vi "Main.vi"(0 "Operations":string(combo), 1 "Delete":bool, 2 "Save":bool, 3 "Load":bool, 5 "Add":bool, 7 "Tree":string(tree), 11 "Error In":errorcluster) -> (15 "Error Out":errorcluster)   [LabVIEW 2023]
doc: "The VI adds the selected the operation into the tree and loads the instances which performs the arithmetic operations and it can save or load the class data into the XML files"
uses:
  Typedef/Queue Operation.ctl
  Typedef/Calculator Data.ctl
  Typedef/Class Data.ctl
  Classes/Arithemtic Operation/Arithemetic Operation.lvclass
  Typedef/DVR Ref.ctl
  Typedef/User Event Operations.ctl
  <vilib>/Utility/xml.llb/Write to XML File(string).vi
  <vilib>/Utility/xml.llb/Read From XML File(array).vi
panel:
  # "Instructions:\n1. Run the VI.\n2. Select the operation to be done from the Operations.\n3. Click Add to create a instance and is added in the tree.\n4. Select the instance name in the tree to load the instance.\n5. Specify the input values in the instance and observe the output\n6. On clicking the Delete button the selected instance will be deleted. \n7. Click Save to save the values all instances in an XML file.\n8. Click Load to load the values of all instances from an XML file.\n9. Click panel close to stop the VI from running."
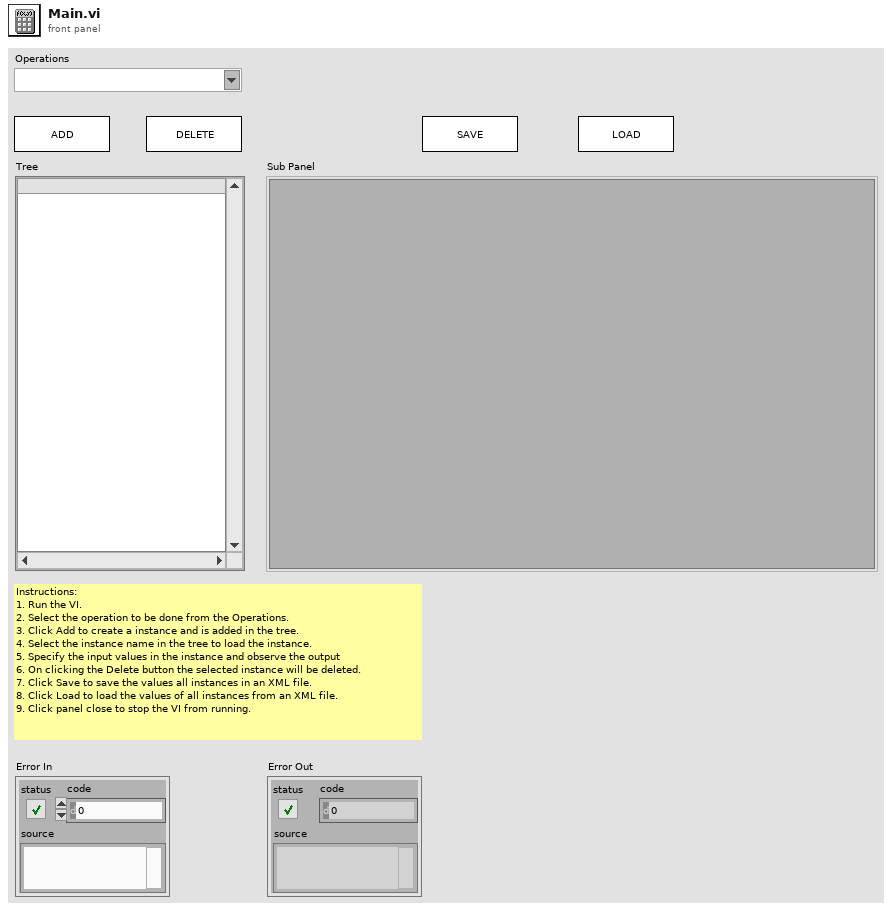
[diagram p1: front panel]
types:
  T1 = typedef "User Event Operations.ctl" = enum16{"Obtain", "Generate", "Release"}
  T2 = typedef "Calculator Data.ctl" = cluster{"Selected Item":string, "Selected Tag":string, "XML Path":path, "Instance Data Array":T3[], "Class Data":refnum<class "Arithemetic Operation.lvclass">, "Class Name":string, "Close":refnum<data-value>, "DVR Ref Array":T4[]}
  T3 = typedef "Class Data.ctl" = cluster{"Class Data":refnum<class "Arithemetic Operation.lvclass">, "Name":string}
  T4 = typedef "DVR Ref.ctl" = cluster{"Class Name":string, "DVR":refnum<data-value>}
  T5 = typedef "Queue Operation.ctl" = enum16{"Create & Enqueue N", "Enqueue N", "Dequeue", "Enstack N", "Flush", "Release"}
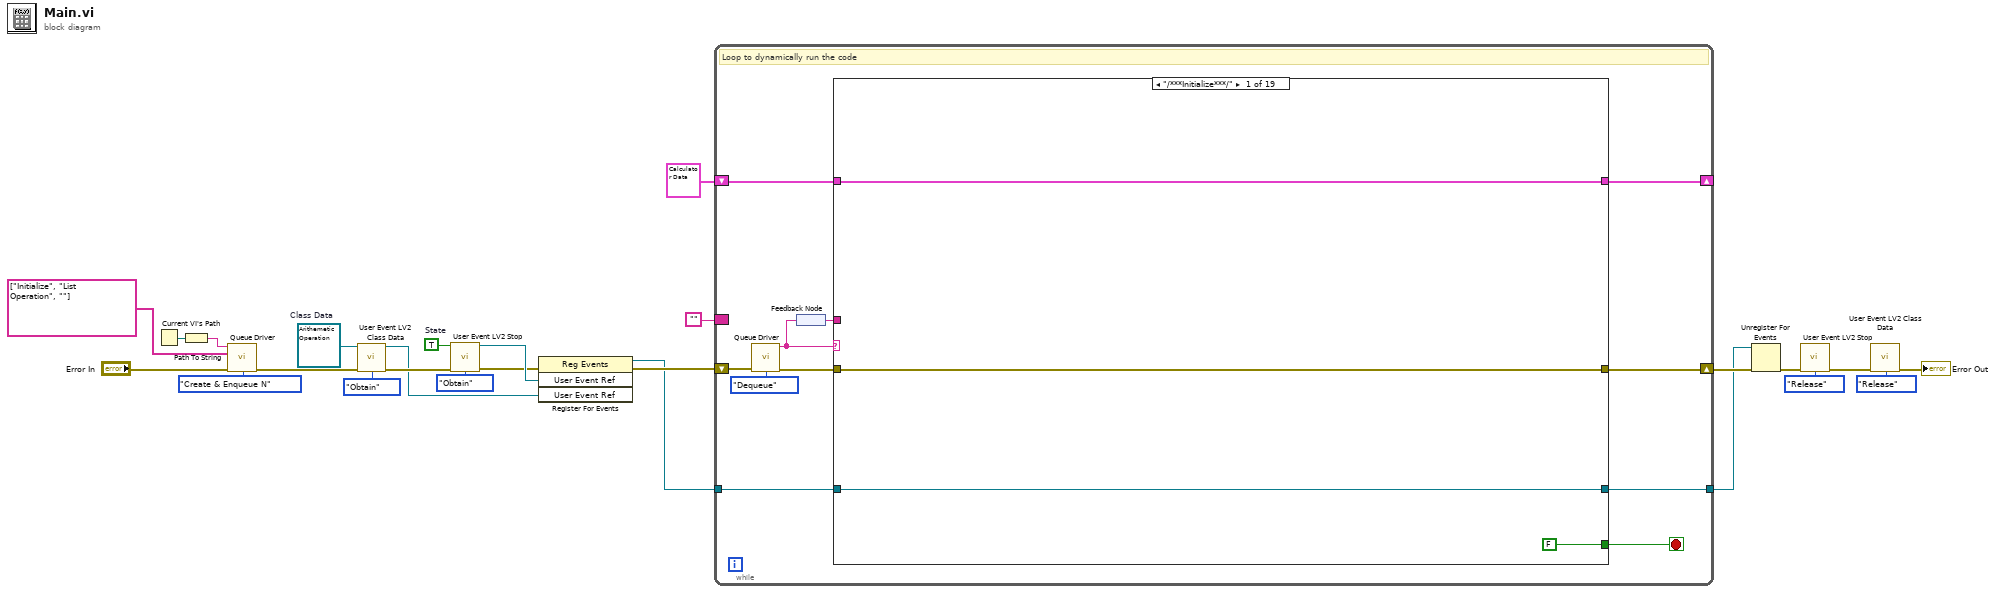
[diagram p0: block diagram]
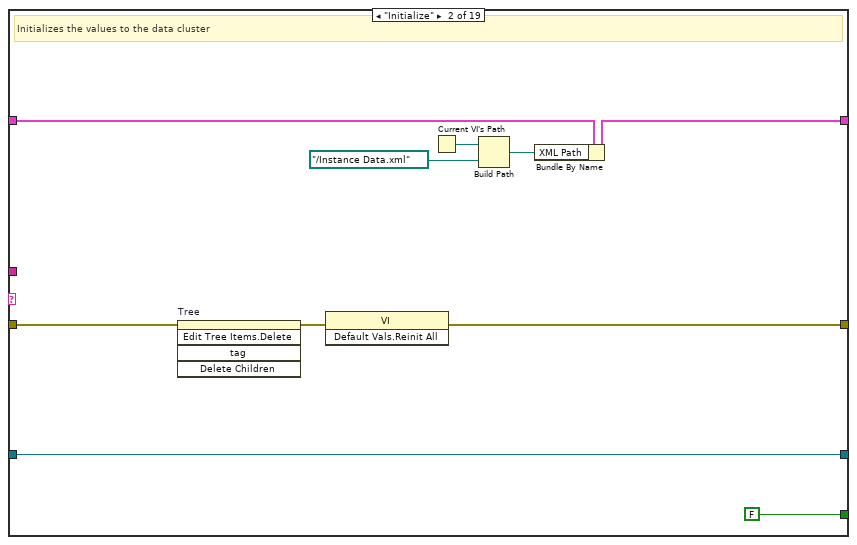
[diagram p2: hidden frame]
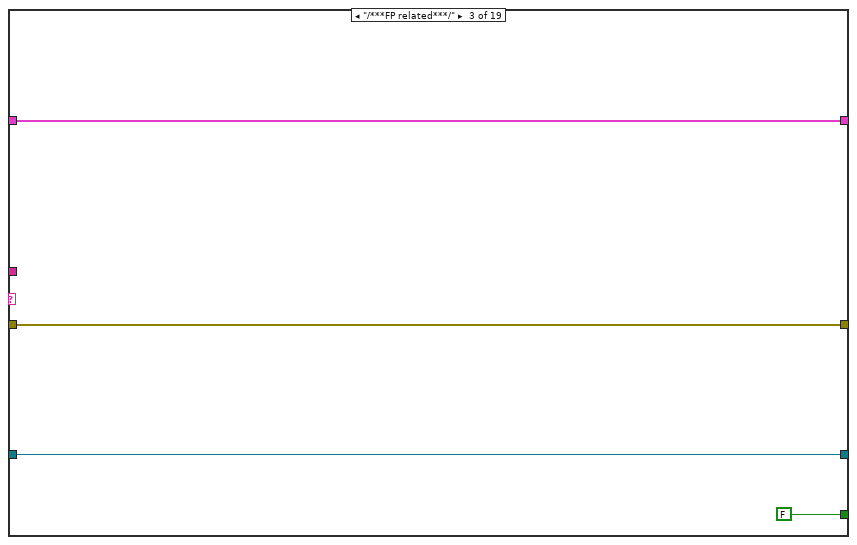
[diagram p3: hidden frame]
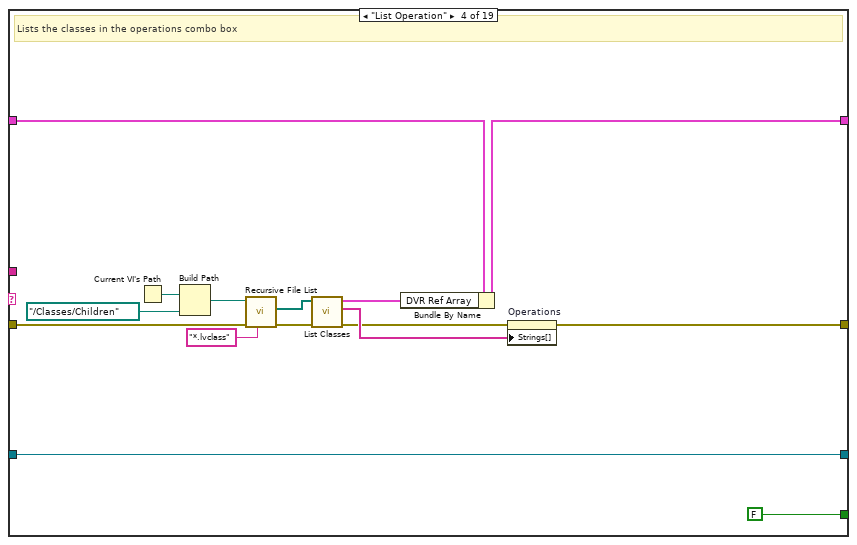
[diagram p4: hidden frame]
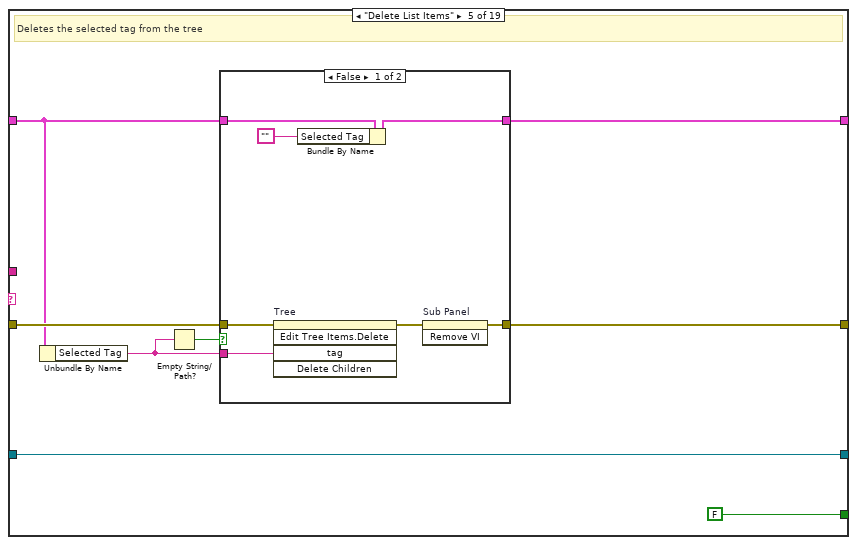
[diagram p5: hidden frame]
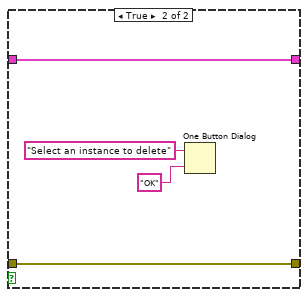
[diagram p6: hidden frame]
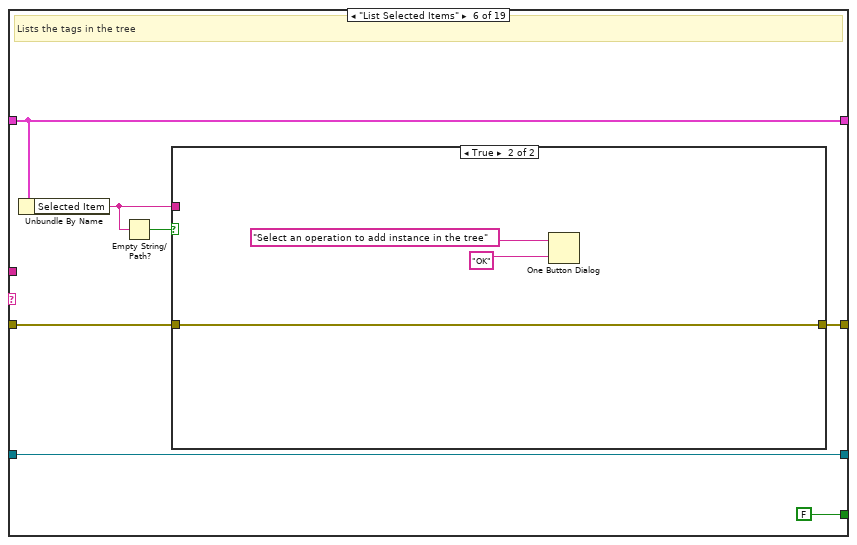
[diagram p7: hidden frame]
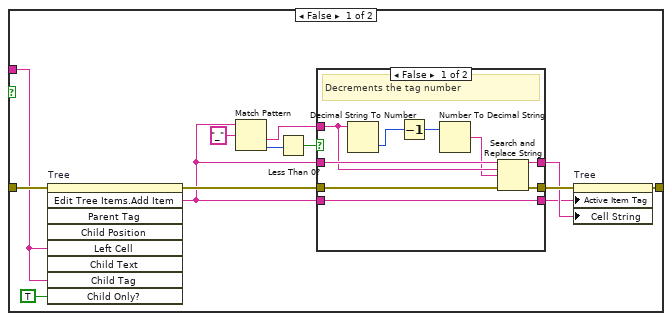
[diagram p8: hidden frame]
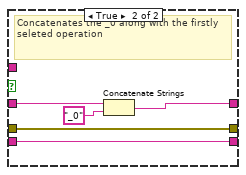
[diagram p9: hidden frame]
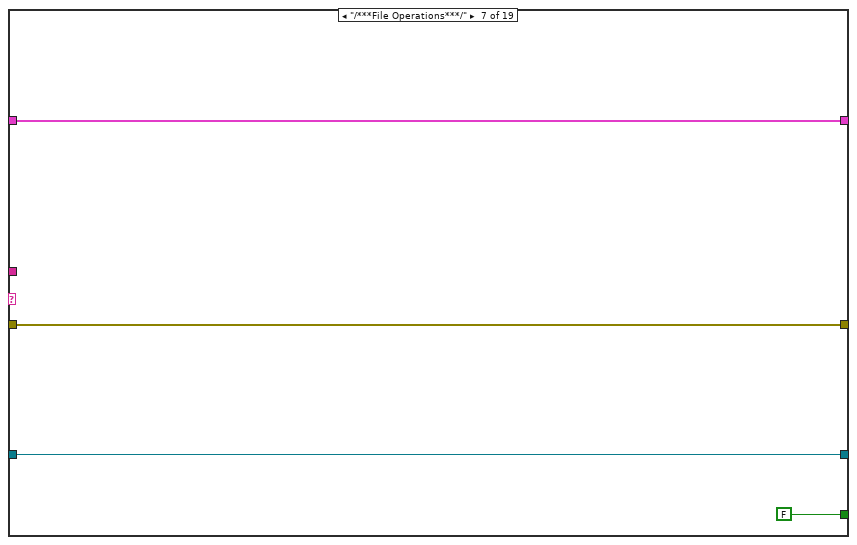
[diagram p10: hidden frame]
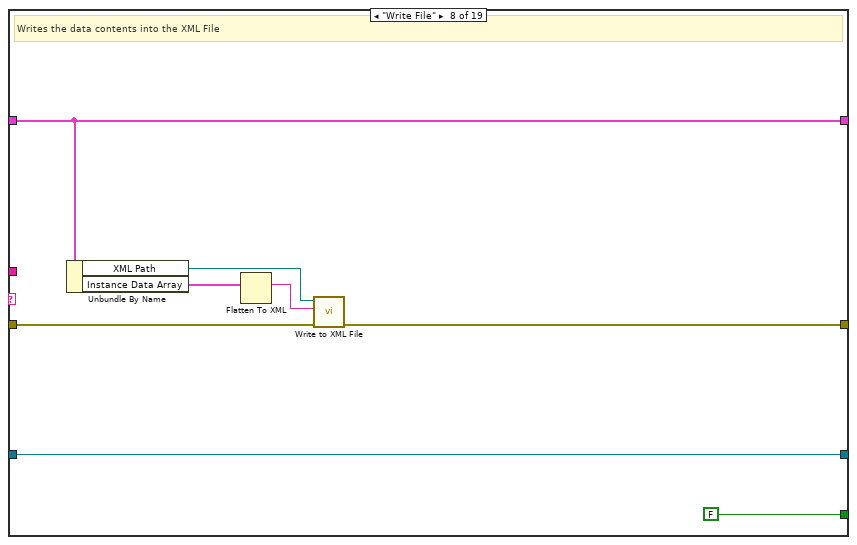
[diagram p11: hidden frame]
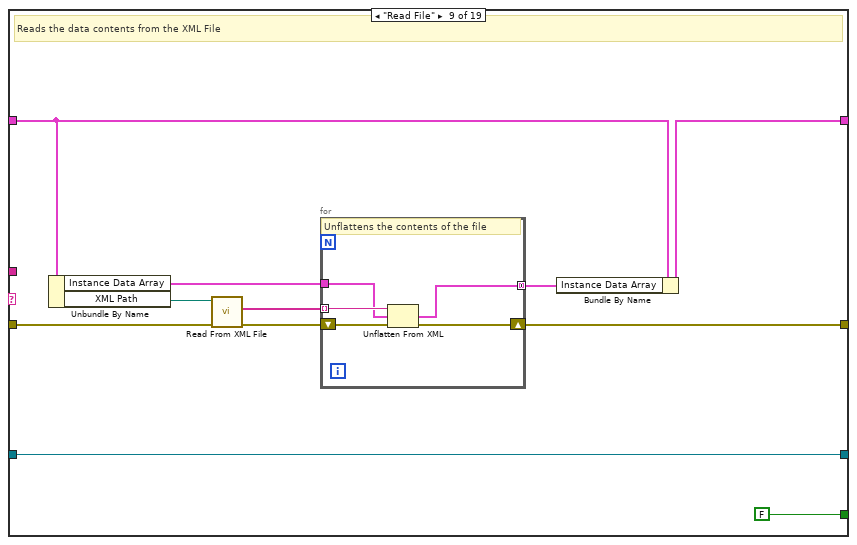
[diagram p12: hidden frame]
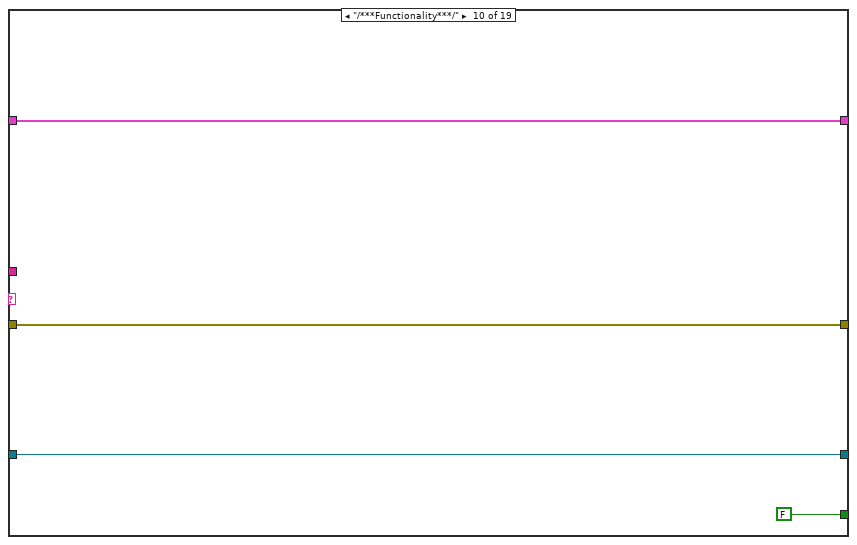
[diagram p13: hidden frame]
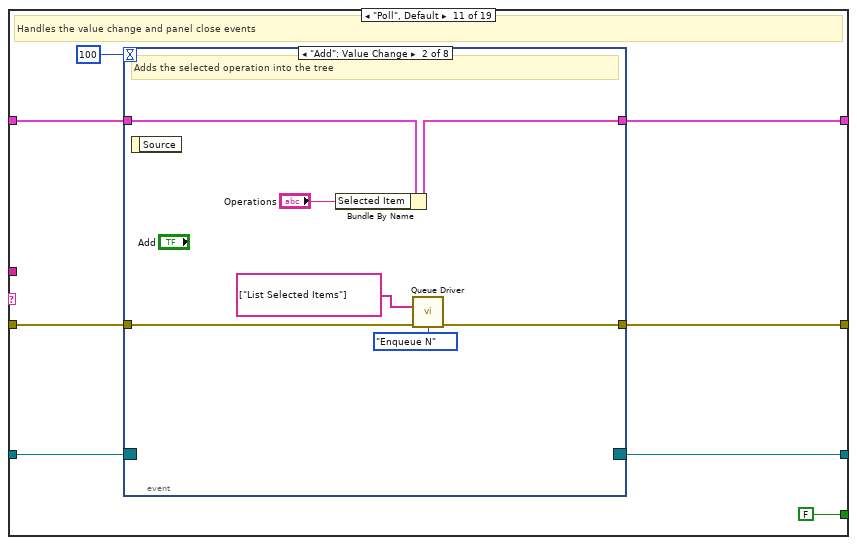
[diagram p14: hidden frame]
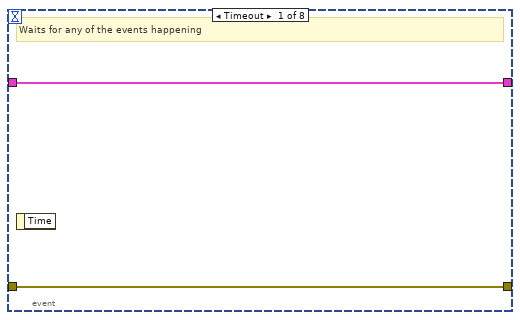
[diagram p15: hidden frame]
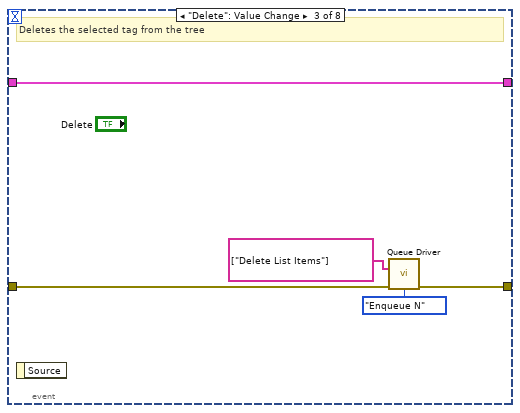
[diagram p16: hidden frame]
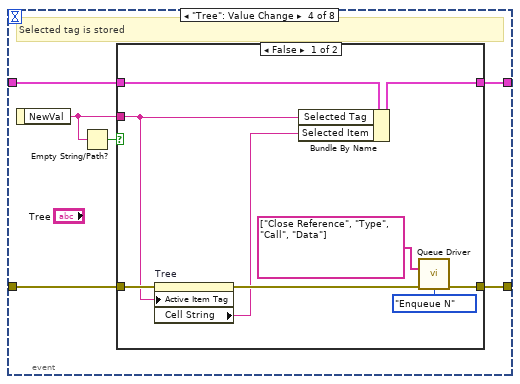
[diagram p17: hidden frame]
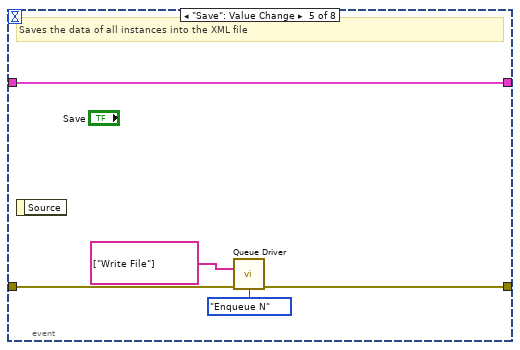
[diagram p19: hidden frame]
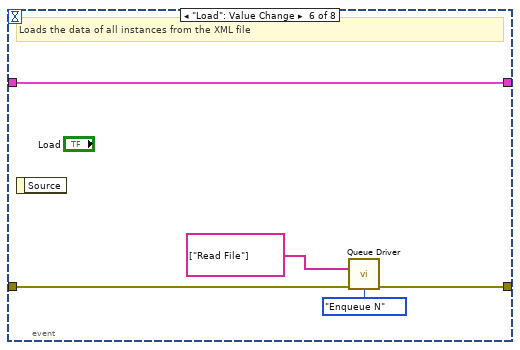
[diagram p20: hidden frame]
diagram:
  w8 = refnum<class "Arithemetic Operation.lvclass"> refnum  # Class Data
  w19 = TRUE  # State
  n1 = Current VI's Path() -> (path=w3:path)
  n2 = Path To String(path=w3) -> (string=w2:string)
  n3 = call "Queue Driver.vi"("Queue Name"=w2, "States[]"=string[] ["Initialize", "List Operation", ""] ("Array of States"), "Error In"="Error In", "Queue Operation"=Queue_Operation."Create & Enqueue N") -> ("Error Out"=w23:errorcluster)  [unwired: 10 in, 1 out]
  n4 = call "User Event LV2 Class Data.vi"("Class Data"=w8, "Error In"=w23, "Operation"=User_Event_Operations."Obtain") -> ("User Event Ref"=w16:refnum<user-event>, "Error Out"=w17:errorcluster)  [unwired: 11 in]
  n5 = call "User Event LV2 Stop.vi"("Stop"=w19, "Error In"=w17, "Operation"=User_Event_Operations."Obtain") -> ("User Event Ref"=w7:refnum<user-event>, "Error Out"=w6:errorcluster)  [unwired: 11 in]
  n6 = register-events(error in=w6, w7, w16) -> (reference out=w15:refnum<event-registration>, error out=w18:errorcluster)  [unwired: 1 in]
  n7 = while {
    shift-right: [w32] -> _
    shift-left: T2 {"Selected Item"="", "Selected Tag"="", "XML Path"=path "", "Instance Data Array"=[], "Class Data"=refnum, "Class Name"="", "Close"=refnum, "DVR Ref Array"=[]} ("Calculator Data") -> [w33]
    border: "" ("Dequeue Element") -> [_]
    shift-right: [w34] -> w22
    shift-left: w18 -> [w36]
    tunnel: w15 -> [w27]
    tunnel: [w26] -> w11
    stop <- w31 stop-if-true
    # "Loop to dynamically run the code"
    n8 = call "Queue Driver.vi"("Error In"=w36, "Queue Operation"=Queue_Operation."Dequeue") -> ("Dequeue Element"=w29:string, "Error Out"=w35:errorcluster)  [unwired: 12 in]
    n9 = feedback-in #1(w29) -> ()
    n10 = feedback #1() -> (w30:string)
    n11 = case shown="\"/***Initialize***/\"" w29 {
      tunnel: w35 -> [w40 w50 w54 w66 w77 w95 w129 w137 w148 w157 w165 w230 w239 w250 w257 w273 w280 w299 w302]
      tunnel: [w40 w41 w54 w64 w74 w92 w129 w134 w147 w157 w164 w227 w237 w250 w259 w273 w282 w299 w303] -> w34
      tunnel: w33 -> [w39 w49 w53 w58 w73 w94 w128 w135 w144 w156 w162 w228 w241 w249 w255 w272 w288 w298 w305]
      tunnel: [w39 w45 w53 w57 w72 w94 w128 w135 w140 w156 w161 w228 w241 w248 w261 w272 w288 w298 w305] -> w32
      tunnel: [FALSE ("Stop") FALSE ("Stop") FALSE ("Stop") FALSE ("Stop") FALSE ("Stop") FALSE ("Stop") FALSE ("Stop") FALSE ("Stop") FALSE ("Stop") FALSE ("Stop") FALSE ("Stop") FALSE ("Stop") FALSE ("Stop") FALSE ("Stop") FALSE ("Stop") FALSE ("Stop") FALSE ("Stop") FALSE ("Stop") TRUE ("Stop")] -> w31
      tunnel: w30 -> [_ _ _ _ _ _ _ _ _ _ _ _ _ _ _ _ w276 _ _]
      tunnel: w27 -> [w38 w46 w52 w69 w75 w91 w127 w131 w138 w155 w159 w229 w236 w247 w263 w271 w274 w297 w300]
      tunnel: [w38 w46 w52 w69 w75 w91 w127 w131 w138 w155 w158 w229 w236 w247 w263 w271 w274 w297 w300] -> w26
      frame "/***Initialize***/" {
      }
      frame "Initialize" {
        # "Initializes the values to the data cluster"
        n12 = invoke on="Tree" class="Tree (strict)" method="Edit Tree Items.Delete"(error in=w50) -> (error out=w47:errorcluster)  [unwired: 4 in, 4 out]
        n13 = invoke class="VI" method="Default Vals.Reinit All"(error in=w47) -> (error out=w41:errorcluster)  [unwired: 2 in, 2 out]
        n14 = Current VI's Path() -> (path=w44:path)
        n15 = Build Path(base path=w44, name or relative path=path "../Instance Data.xml") -> (appended path=w42:path)
        n16 = Bundle By Name(cluster=w49, "XML Path"=w42) -> (w45:T2)
      }
      frame "/***FP related***/" {
      }
      frame "List Operation" {
        # "Lists the classes in the operations combo box"
        n17 = Current VI's Path() -> (path=w68:path)
        n18 = Build Path(base path=w68, name or relative path=path "../Classes/Children") -> (appended path=w65:path)
        n19 = call <vilib>:"Recursive File List.vi"("pattern"="*.lvclass", "error in (no error)"=w66, "Folder Path"=w65) -> ("error out"=w60:errorcluster, "All Files in Dir"=w55:path[])  [unwired: 4 in, 3 out]
        n20 = call "List Classes.vi"("Error In"=w60, "Class Path"=w55) -> ("Error Out"=w59:errorcluster, "Class Names"=w63:string[], "DVR Ref"=w56:T4[])  [unwired: 7 in]
        n21 = Bundle By Name(cluster=w58, "DVR Ref Array"=w56) -> (w57:T2)
        n22 = property on="Operations" class="CmbBox"(error in=w59, "Strings[]"=w63) -> (error out=w64:errorcluster)  [unwired: 1 in, 1 out]
      }
      frame "Delete List Items" {
        # "Deletes the selected tag from the tree"
        n23 = Unbundle By Name(w73) -> ("Selected Tag"=w71:string)
        n24 = Empty String/Path?(string/path=w71) -> (empty?=w70:bool)
        n25 = case shown="False" w70 {
          tunnel: w77 -> [w84 w87]
          tunnel: w71 -> [w82 _]
          tunnel: [w81 w87] -> w74
          tunnel: w73 -> [w80 w88]
          tunnel: [w79 w88] -> w72
          frame False {
            n26 = invoke on="Tree" class="Tree (strict)" method="Edit Tree Items.Delete"(error in=w84, "tag"=w82) -> (error out=w83:errorcluster)  [unwired: 3 in, 4 out]
            n27 = Bundle By Name(cluster=w80, "Selected Tag"="") -> (w79:T2)
            n28 = invoke on="Sub Panel" class="SubPnl" method="Remove VI"(error in=w83) -> (error out=w81:errorcluster)  [unwired: 2 in, 2 out]
          }
          frame True {
            n29 = One Button Dialog(message="Select an instance to delete", button name ("OK")="OK") -> ()  [unwired: 1 out]
          }
        }
      }
      frame "List Selected Items" {
        # "Lists the tags in the tree"
        n30 = Unbundle By Name(w94) -> ("Selected Item"=w89:string)
        n31 = Empty String/Path?(string/path=w89) -> (empty?=w90:bool)
        n32 = case shown="True" w90 {
          tunnel: w95 -> [w108 w125]
          tunnel: w89 -> [w96 _]
          tunnel: [w101 w125] -> w92
          frame False {
            n33 = invoke on="Tree" class="Tree (strict)" method="Edit Tree Items.Add Item"(error in=w108, "Left Cell"=w96, "Child Tag"=w96, "Child Only?"=TRUE) -> (error out=w106:errorcluster, "Edit Tree Items:Add Item"=w99:string)  [unwired: 5 in, 7 out]
            n34 = Match Pattern(string=w99, regular expression="_") -> (after substring=w102:string, offset past match=w105:i32)  [unwired: 1 in, 2 out]
            n35 = Less Than 0?(x=w105) -> (x < 0?=w103:bool)
            n36 = case shown="False" w103 {
              tunnel: w106 -> [w117 w122]
              tunnel: [w116 w122] -> w104
              tunnel: w99 -> [w115 w121]
              tunnel: w102 -> [w114 _]
              tunnel: [w111 w119] -> w100
              tunnel: w99 -> [w109 w118]
              tunnel: [w109 w118] -> w98
              frame False {
                # "Decrements the tag number"
                n37 = Decimal String To Number(string=w114) -> (number=w110:i32)  [unwired: 2 in, 1 out]
                n38 = Decrement(x=w110) -> (x-1=w113:i32)
                n39 = Number To Decimal String(number=w113) -> (decimal integer string=w112:string)  [unwired: 1 in]
                n40 = Search and Replace String(input string=w115, search string=w114, replace string=w112, error in=w117) -> (result string=w111:string, error out=w116:errorcluster)  [unwired: 4 in, 2 out]
              }
              frame True {
                # "Concatenates the _0 along with the firstly seleted operation"
                n41 = Concatenate Strings(w121, "_0" ("string")) -> (w119:string)
              }
            }
            n42 = property on="Tree" class="Tree (strict)"(error in=w104, "Active Item Tag"=w98, "Cell String"=w100) -> (error out=w101:errorcluster)  [unwired: 1 in, 1 out]
          }
          frame True {
            n43 = One Button Dialog(message="Select an operation to add instance in the tree", button name ("OK")="OK") -> ()  [unwired: 1 out]
          }
        }
      }
      frame "/***File Operations***/" {
      }
      frame "Write File" {
        # "Writes the data contents into the XML File"
        n44 = Unbundle By Name(w135) -> ("XML Path"=w130:path, "Instance Data Array"=w133:T3[])
        n45 = Flatten To XML(6:w133) -> (2:w132:string)
        n46 = call-poly <vilib>:"Write to XML File.vi"("error in (no error)"=w137, "XML Input"=w132, "XML File Path"=w130) -> ("error out"=w134:errorcluster)  [unwired: 6 in, 2 out]
      }
      frame "Read File" {
        # "Reads the data contents from the XML File"
        n47 = Unbundle By Name(w144) -> ("Instance Data Array"=w141:T3[], "XML Path"=w143:path)
        n48 = call-poly <vilib>:"Read From XML File.vi"("error in (no error)"=w148, "XML File Path"=w143) -> ("error out"=w145:errorcluster, "XML Elements"=w142:string[])  [unwired: 7 in, 1 out]
        n49 = for {
          tunnel: w142 -> [w151] mode=indexing
          shift-right: [w153] -> w147
          shift-left: w145 -> [w152]
          tunnel: w141 -> [w150]
          tunnel: [w149] -> w139 mode=concatenating
          # "Unflattens the contents of the file"
          n50 = Unflatten From XML(xml string=w151, type=w150, error in (no error)=w152) -> (value=w149:T3[], error out=w153:errorcluster)
        }
        n51 = Bundle By Name(cluster=w144, "Instance Data Array"=w139) -> (w140:T2)
      }
      frame "/***Functionality***/" {
      }
      frame "Poll", Default {
        # "Handles the value change and panel close events"
        n52 = event shown="[1] \"Add\": Value Change" {
          selector: w159 -> [_ _ _ _ _ _ _ _]
          dyn-events: [_ _ _ _ _ _ _ _] -> w158
          timeout: 100 -> [_ _ _ _ _ _ _ _]
          tunnel: w165 -> [w167 w172 w179 w185 w199 w204 w215 w217]
          tunnel: [w167 w171 w178 w182 w198 w203 w210 w216] -> w164
          tunnel: w162 -> [w166 w174 w177 w184 w201 w206 w214 w223]
          tunnel: [w166 w170 w177 w183 w201 w206 w214 w219] -> w161
          event Timeout {
            # "Waits for any of the events happening"
            n53 = event-data() -> ()  [unwired: 1 in, 1 out]
          }
          event "Add": Value Change {
            # "Adds the selected operation into the tree"
            n54 = event-data() -> ()  [unwired: 1 in, 1 out]
            n55 = Bundle By Name(cluster=w174, "Selected Item"="Operations") -> (w170:T2)
            n56 = call "Queue Driver.vi"("States[]"=string[] ["List Selected Items"] ("Array of States"), "Error In"=w172, "Queue Operation"=Queue_Operation."Enqueue N") -> ("Error Out"=w171:errorcluster)  [unwired: 11 in, 1 out]
          }
          event "Delete": Value Change {
            # "Deletes the selected tag from the tree"
            n57 = event-data() -> ()  [unwired: 1 in, 1 out]
            n58 = call "Queue Driver.vi"("States[]"=string[] ["Delete List Items"] ("Array of States"), "Error In"=w179, "Queue Operation"=Queue_Operation."Enqueue N") -> ("Error Out"=w178:errorcluster)  [unwired: 11 in, 1 out]
          }
          event "Tree": Value Change {
            # "Selected tag is stored"
            n59 = event-data() -> ("NewVal"=w180:string)  [unwired: 1 in]
            n60 = Empty String/Path?(string/path=w180) -> (empty?=w181:bool)
            n61 = case shown="False" w181 {
              tunnel: w185 -> [w194 w195]
              tunnel: w184 -> [w193 w196]
              tunnel: [w192 w196] -> w183
              tunnel: [w191 w195] -> w182
              tunnel: w180 -> [w186 _]
              frame False {
                n62 = property on="Tree" class="Tree (strict)"(error in=w194, "Active Item Tag"=w186) -> (error out=w188:errorcluster, "Cell String"=w187:string)  [unwired: 1 in, 1 out]
                n63 = Bundle By Name(cluster=w193, "Selected Tag"=w186, "Selected Item"=w187) -> (w192:T2)
                n64 = call "Queue Driver.vi"("States[]"=string[] ["Close Reference", "Type", "Call", "Data"] ("Array of States"), "Error In"=w188, "Queue Operation"=Queue_Operation."Enqueue N") -> ("Error Out"=w191:errorcluster)  [unwired: 11 in, 1 out]
              }
              frame True {
              }
            }
          }
          event "Save": Value Change {
            # "Saves the data of all instances into the XML file"
            n65 = event-data() -> ()  [unwired: 1 in, 1 out]
            n66 = call "Queue Driver.vi"("States[]"=string[] ["Write File"] ("Array of States"), "Error In"=w199, "Queue Operation"=Queue_Operation."Enqueue N") -> ("Error Out"=w198:errorcluster)  [unwired: 11 in, 1 out]
          }
          event "Load": Value Change {
            # "Loads the data of all instances from the XML file"
            n67 = event-data() -> ()  [unwired: 1 in, 1 out]
            n68 = call "Queue Driver.vi"("States[]"=string[] ["Read File"] ("Array of States"), "Error In"=w204, "Queue Operation"=Queue_Operation."Enqueue N") -> ("Error Out"=w203:errorcluster)  [unwired: 11 in, 1 out]
          }
          event Panel Close? {
            w209 = TRUE  # State
            # "Enqueues the exit state to stop the VI running"
            n69 = event-data() -> ()  [unwired: 1 in, 1 out]
            n70 = call "Queue Driver.vi"("States[]"=string[] ["Exit"] ("Array of States"), "Error In"=w215, "Queue Operation"=Queue_Operation."Enqueue N") -> ("Error Out"=w212:errorcluster)  [unwired: 11 in, 1 out]
            n71 = call "User Event LV2 Stop.vi"("Stop"=w209, "Error In"=w212, "Operation"=User_Event_Operations."Generate") -> ("Error Out"=w210:errorcluster)  [unwired: 11 in, 1 out]
            n72 = event-data("Discard?"=TRUE) -> ()  [unwired: 1 in, 1 out]
          }
          event User Event {
            # "Stores the instance data"
            n73 = event-data() -> ("Arithemetic Operation.lvclass"=w222:refnum<class "Arithemetic Operation.lvclass">)  [unwired: 1 in]
            n74 = Unbundle By Name(w223) -> ("Instance Data Array"=w221:T3[], "Selected Item"=w220:string)
            n75 = call "Instance History.vi"("Instance Data Array in"=w221, "Selected Instance"=w220, "Class Data"=w222, "Error In"=w217) -> ("Instance Data Array out"=w218:T3[], "Error Out"=w216:errorcluster)  [unwired: 5 in]
            n76 = Bundle By Name(cluster=w223, "Instance Data Array"=w218) -> (w219:T2)
          }
        }
      }
      frame "Close Reference" {
        # "Closes the asynchronous call reference of the previous instance"
        n77 = Unbundle By Name(w228) -> ("Close"=w224:refnum<data-value>)
        n78 = Not A Number/Path/Refnum?(number/path/refnum=w224) -> (NaN/Path/Refnum?=w225:bool)
        n79 = case shown="False" w225 {
          tunnel: w230 -> [w233 w234]
          tunnel: [w232 w234] -> w227
          tunnel: w224 -> [w231 _]
          frame False {
            # "Close the VI reference"
            n80 = call "Close Ref.vi"("Error In"=w233, "DVR Ref"=w231) -> ("Error Out"=w232:errorcluster)  [unwired: 9 in]
          }
          frame True {
          }
        }
      }
      frame "Data" {
        # "Loads the class data for the selected instance"
        n81 = Unbundle By Name(w241) -> ("Instance Data Array"=w240:T3[], "Selected Item"=w235:string)
        n82 = call "get Class Data.vi"("Error In"=w239, "Selected Instance"=w235, "Instance Data Array"=w240) -> ("Error Out"=w237:errorcluster)  [unwired: 8 in]
      }
      frame "Type" {
        # "Updates the class name based on the selected tag"
        n83 = Unbundle By Name(w249) -> ("Selected Tag"=w246:string)
        n84 = Match Pattern(string=w246, regular expression="_") -> (before substring=w244:string)  [unwired: 1 in, 3 out]
        n85 = Concatenate Strings(w244, ".lvclass" ("string")) -> (w242:string)
        n86 = Bundle By Name(cluster=w249, "Class Name"=w242) -> (w248:T2)
      }
      frame "Call" {
        # "Calls the selected operation UI"
        n87 = Unbundle By Name(w255) -> ("DVR Ref Array"=w252:T4[], "Class Name"=w254:string)
        n88 = for {
          shift-right: [w269] -> w256
          shift-left: w257 -> [w269]
          tunnel: w252 -> [w265] mode=indexing
          tunnel: w254 -> [w268]
          tunnel: [w267] -> w253 if=w266
          stop <- w266 stop-if-true
          n89 = Unbundle By Name(w265) -> ("DVR"=w267:refnum<data-value>, "Class Name"=w264:string)
          n90 = Equal?(x=w264, y=w268) -> (x = y?=w266:bool)
        }
        n91 = control-ref of="Sub Panel"() -> (w260:refnum<vi>)
        n92 = call "Caller DVR.vi"("DVR In"=w253, "Sub Panel"=w260, "Error In"=w256) -> ("DVR Out"=w258:refnum<data-value>, "Error Out"=w259:errorcluster)  [unwired: 11 in]
        n93 = Bundle By Name(cluster=w255, "Close"=w258) -> (w261:T2)
      }
      frame "/***Error***/" {
      }
      frame "Error" {
        # "Displays the error encountered and acts according to user acknowledgement"
        n94 = Unbundle By Name(w280) -> ("code"=w279:i32, "source"=w278:string)
        n95 = call <vilib>:"Clear Errors.vi"("error in (no error)"=w280) -> ("error out"=w285:errorcluster)  [unwired: 5 in, 1 out]
        n96 = Format Into String(format string="Error occurred in state \"%s\"!!\nError Code: %d\nError Source: %s\n\nDo you wish to continue?", error in=w285, w276, w279, w278) -> (resulting string=w286:string, error out=w281:errorcluster)  [unwired: 1 in]
        n97 = Two Button Dialog(message=w286, 1:"Exit" ("F button name (\"Cancel\")"), 2:"Continue" ("T button name (\"OK\")")) -> (T button?=w287:bool)
        n98 = case "Continue?" shown="False" w287 {
          tunnel: [w294 w295] -> w282
          tunnel: w281 -> [w291 w295]
          frame False {
            # "Enqueues the exit state to stop the VI running"
            n99 = call "Queue Driver.vi"("Error In"=w291, "Queue Operation"=Queue_Operation."Flush") -> ("Error Out"=w290:errorcluster)  [unwired: 12 in, 1 out]
            n100 = call "Queue Driver.vi"("States[]"=string[] ["Exit"] ("Array of States"), "Error In"=w290, "Queue Operation"=Queue_Operation."Enqueue N") -> ("Error Out"=w294:errorcluster)  [unwired: 11 in, 1 out]
          }
          frame True {
            # "Continues the VI running"
          }
        }
      }
      frame "/***Exit***/" {
      }
      frame "Exit" {
        # "Stops the VI running"
        n101 = call "Queue Driver.vi"("Error In"=w302, "Queue Operation"=Queue_Operation."Release") -> ("Error Out"=w303:errorcluster)  [unwired: 12 in, 1 out]
      }
    }
  }
  n102 = Unregister For Events(event registration refnum=w11, error in=w22) -> (error out=w14:errorcluster)
  n103 = call "User Event LV2 Stop.vi"("Error In"=w14, "Operation"=User_Event_Operations."Release") -> ("Error Out"=w13:errorcluster)  [unwired: 12 in, 1 out]
  n104 = call "User Event LV2 Class Data.vi"("Error In"=w13, "Operation"=User_Event_Operations."Release") -> ("Error Out"=→"Error Out":errorcluster)  [unwired: 12 in, 1 out]
